vi "FGV_HoldingRegs.vi"(6 "FGV_enum":T3=enum."Read", 7 "unit ID":u8=1, 8 "error in (no error)":errorcluster, 9 "FGV_ data cluster":T1={"demux1_10(x6)_encode"=enum."demux1_10_channel0", "mux10_1(x6)_encode"=enum."mux10_1_channel0", "MB Relay01"=[FALSE, FALSE, FALSE, FALSE, FALSE, FALSE], "SpareRelays (DPDT)"=[], "mux6_1(3wires)_encode"=enum."mux6-1_channel0", "mux2-1(DMM I) encode"=enum."DMM I (0.5)", "5V enable"=FALSE, "SpareRelays (SPDT)"=[FALSE, FALSE, FALSE, FALSE, FALSE, FALSE, FALSE, FALSE, FALSE, FALSE, FALSE, FALSE, FALSE, FALSE, FALSE, FALSE, FALSE, FALSE, FALSE, FALSE, FALSE, FALSE, FALSE, FALSE, FALSE, FALSE, FALSE, FALSE, FALSE, FALSE, FALSE, FALSE], "JIG_RESET"=FALSE}, 10 "Instruments":T2=enum."mux10_1(x6)", 11 "Modbus master in":refnum<class "Modbus Master.lvclass">) -> (0 "error out":errorcluster, 2 "HoldingRegs":u16[](array[numeric]), 3 "Modbus master out":refnum<class "Modbus Master.lvclass">)   [LabVIEW 2018, in "MB Relay.lvlib"]
uses:
  MB Relay.lvlib
  type defs/FGV enum.ctl
  <vilib>/NI/Modbus Library/API/Master/Modbus Master.lvclass
  C:/Program Files (x86)/National Instruments/LabVIEW 2018/vi.lib/NI/Modbus Library/API/Modbus API.lvclass
  type defs/MB relays _InstrumentType.ctl
  type defs/FGV data cluster.ctl
  <vilib>/NI/Modbus Library/API/Modbus API.lvclass/Modbus API.ctl
  <vilib>/NI/Modbus Library/Transmission Data Unit/Transmission Data Unit.lvclass/Transmission Data Unit.ctl
  <vilib>/NI/Modbus Library/Transmission Data Unit/Write Unit ID.vi
  <vilib>/NI/Modbus Library/API/Read Transmission Data Unit.vi
  <vilib>/NI/Modbus Library/API/Write Transmission Data Unit.vi
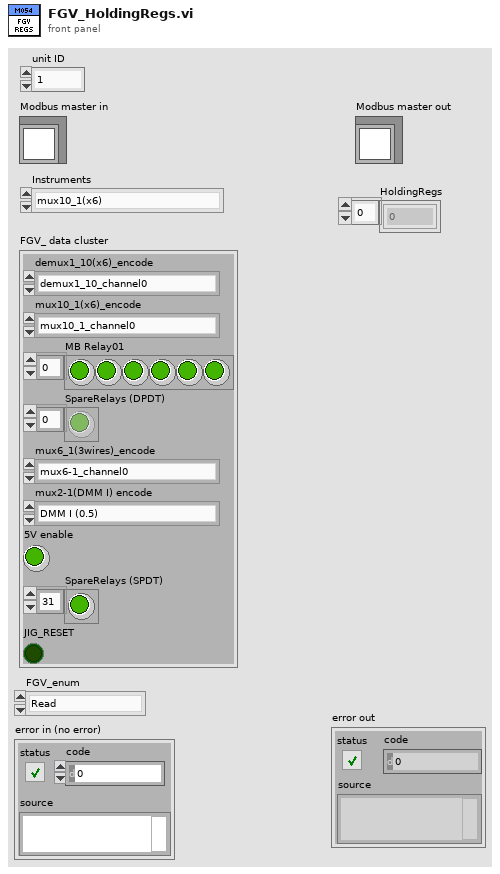
[diagram p1: front panel]
types:
  T1 = typedef "MB Relay.lvlib/FGV data cluster.ctl" = cluster{"demux1_10(x6)_encode":enum16{"demux1_10_channel0", "demux1_10_channel1", "demux1_10_channel2", "demux1_10_channel3", "demux1_10_channel4", "demux1_10_channel5", "demux1_10_channel6", "demux1_10_channel7", "demux1_10_channel8", "demux1_10_channel9", "demux1_10_channel10"}, "mux10_1(x6)_encode":enum16{"mux10_1_channel0", "mux10_1_channel1", "mux10_1_channel2", "mux10_1_channel3", "mux10_1_channel4", "mux10_1_channel5", "mux10_1_channel6", "mux10_1_channel7", "mux10_1_channel8", "mux10_1_channel9", "mux10_1_channel10"}, "MB Relay01":bool[], "SpareRelays (DPDT)":bool[], "mux6_1(3wires)_encode":enum16{"mux6-1_channel0", "mux6_1_channel1_0", "mux6_1_channel1_1", "mux6-1_channel1_2", "mux6_1_channel1_3", "mux6_1_channel2_0", "mux6_1_channel2_1", "mux6_1_channel2_2", "mux6_1_channel2_3", "mux6_1_channel3_0", "mux6_1_channel3_1", "mux6_1_channel3_2", "mux6_1_channel3_3", "mux6_1_channel4_0", "mux6_1_channel4_1", "mux6_1_channel4_2", "mux6_1_channel4_3", "mux6_1_channel5_0", "mux6_1_channel5_1", "mux6_1_channel5_2", "mux6_1_channel5_3", "mux6_1_channel6_0", "mux6_1_channel6_1", "mux6_1_channel6_2", "mux6_1_channel6_3"}, "mux2-1(DMM I) encode":enum16{"DMM I (0.5)", "DMM I (12)"}, "5V enable":bool, "SpareRelays (SPDT)":bool[], "JIG_RESET":bool}
  T2 = typedef "MB Relay.lvlib/MB relays _InstrumentType.ctl" = enum16{"JIG_TRIGGER", "JIG_RESET", "Relay SelfTest", "counter", "demux1_10(x6)", "mux10_1(x6)", "mux6_1(3wires)", "MB_Relay_01(eMICs)", "SpareRelays(DPDT)", "Optos", "Inputs", "DMM I 0.5", "SpareRelays (SPDT)", "SC enable"}
  T3 = typedef "MB Relay.lvlib/FGV enum.ctl" = enum16{"Write", "Init FGV", "Read", "All OFF", "All ON"}
  T4 = enum16{"demux1_10_channel0", "demux1_10_channel1", "demux1_10_channel2", "demux1_10_channel3", "demux1_10_channel4", "demux1_10_channel5", "demux1_10_channel6", "demux1_10_channel7", "demux1_10_channel8", "demux1_10_channel9", "demux1_10_channel10"}
  T5 = enum16{"mux10_1_channel0", "mux10_1_channel1", "mux10_1_channel2", "mux10_1_channel3", "mux10_1_channel4", "mux10_1_channel5", "mux10_1_channel6", "mux10_1_channel7", "mux10_1_channel8", "mux10_1_channel9", "mux10_1_channel10"}
  T6 = enum16{"mux6-1_channel0", "mux6_1_channel1_0", "mux6_1_channel1_1", "mux6-1_channel1_2", "mux6_1_channel1_3", "mux6_1_channel2_0", "mux6_1_channel2_1", "mux6_1_channel2_2", "mux6_1_channel2_3", "mux6_1_channel3_0", "mux6_1_channel3_1", "mux6_1_channel3_2", "mux6_1_channel3_3", "mux6_1_channel4_0", "mux6_1_channel4_1", "mux6_1_channel4_2", "mux6_1_channel4_3", "mux6_1_channel5_0", "mux6_1_channel5_1", "mux6_1_channel5_2", "mux6_1_channel5_3", "mux6_1_channel6_0", "mux6_1_channel6_1", "mux6_1_channel6_2", "mux6_1_channel6_3"}
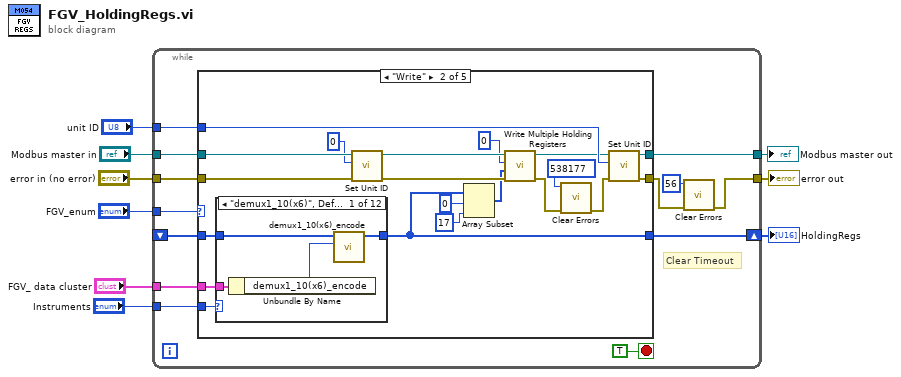
[diagram p0: block diagram]
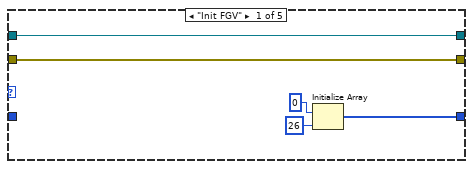
[diagram p2: hidden frame]
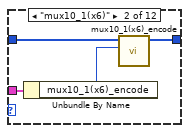
[diagram p3: hidden frame]
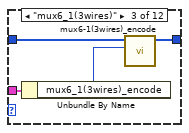
[diagram p4: hidden frame]
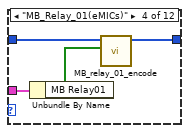
[diagram p5: hidden frame]
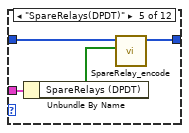
[diagram p6: hidden frame]
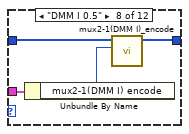
[diagram p9: hidden frame]
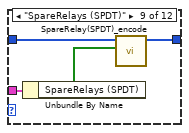
[diagram p10: hidden frame]
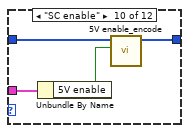
[diagram p11: hidden frame]
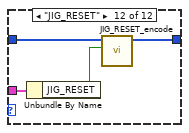
[diagram p13: hidden frame]
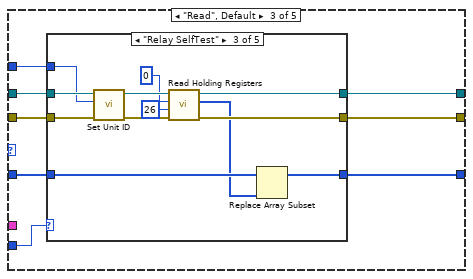
[diagram p14: hidden frame]
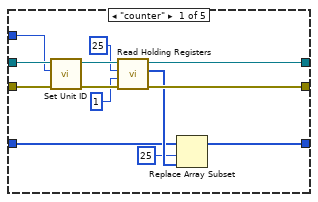
[diagram p15: hidden frame]
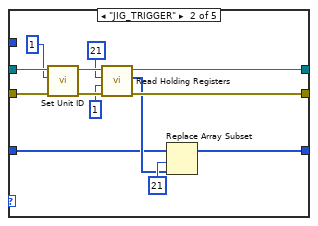
[diagram p16: hidden frame]
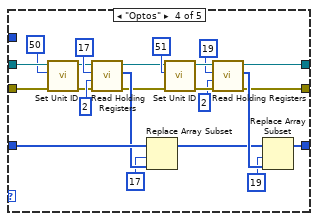
[diagram p17: hidden frame]
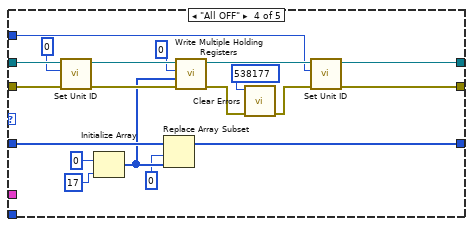
[diagram p19: hidden frame]
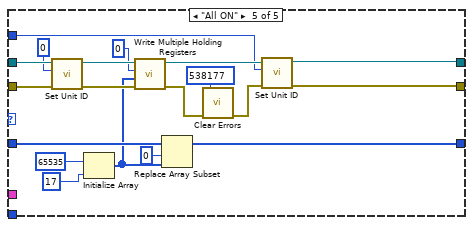
[diagram p20: hidden frame]
diagram:
  n1 = while {
    tunnel: "FGV_enum" -> [w21]
    shift-right: [w20] -> w4
    shift-left: _ -> [w11]
    tunnel: "error in (no error)" -> [w19]
    tunnel: [w14] -> w7
    tunnel: "Modbus master in" -> [w18]
    tunnel: [w17] -> w5
    tunnel: "unit ID" -> [w16]
    tunnel: "Instruments" -> [w12]
    tunnel: "FGV_ data cluster" -> [w10]
    stop <- TRUE stop-if-true
    # "Clear Timeout"
    n2 = case shown="\"Write\"" w21 {
      tunnel: [w24 w31 w91 w161 w184] -> w20
      tunnel: w19 -> [w27 w47 w94 w177 w194]
      tunnel: [w27 w37 w90 w166 w182] -> w15
      tunnel: w18 -> [w23 w44 w93 w175 w192]
      tunnel: [w23 w39 w89 w165 w180] -> w17
      tunnel: w16 -> [_ w36 w87 w164 w179]
      tunnel: w12 -> [_ w32 w88 _ _]
      tunnel: w11 -> [_ w29 w92 w163 w186]
      tunnel: w10 -> [_ w28 _ _ _]
      frame "Init FGV" {
        n3 = Initialize Array(u16 0, 26 ("dimension size")) -> (w24:u16[])
      }
      frame "Write" {
        n4 = case shown="\"demux1_10(x6)\", Default" w32 {
          tunnel: w29 -> [w51 w55 w57 w63 w67 w68 w69 w73 w77 w78 w82 w86]
          tunnel: [w50 w54 w58 w62 w66 w68 w69 w72 w76 w79 w82 w85] -> w31
          tunnel: w28 -> [w49 w53 w59 w61 w65 _ _ w71 w75 w81 _ w84]
          frame "demux1_10(x6)", Default {
            n5 = Unbundle By Name(w49) -> ("demux1_10(x6)_encode"=w48:T4)
            n6 = call "demux1_10(x6)_encode.vi"("demux1_10(x6)_encode"=w48, "Mem_mapping in"=w51) -> ("MemMapping Out"=w50:u16[])  [unwired: 8 in, 1 out]
          }
          frame "mux10_1(x6)" {
            n7 = Unbundle By Name(w53) -> ("mux10_1(x6)_encode"=w52:T5)
            n8 = call "mux10_1(x6)_encode.vi"("mux10_1(x6)_encode"=w52, "Mem_mapping in"=w55) -> ("MemMapping Out"=w54:u16[])  [unwired: 8 in, 1 out]
          }
          frame "mux6_1(3wires)" {
            n9 = Unbundle By Name(w59) -> ("mux6_1(3wires)_encode"=w56:T6)
            n10 = call "mux6-1(3wires)_encode.vi"("mux6_1(3wires)_encode"=w56, "Mem_mapping in"=w57) -> ("MemMapping Out"=w58:u16[])  [unwired: 8 in, 1 out]
          }
          frame "MB_Relay_01(eMICs)" {
            n11 = Unbundle By Name(w61) -> ("MB Relay01"=w60:bool[])
            n12 = call "MB_relay_01_encode.vi"("eMic1-6"=w60, "Mem_mapping in"=w63) -> ("MemMapping Out"=w62:u16[])  [unwired: 8 in, 1 out]
          }
          frame "SpareRelays(DPDT)" {
            n13 = Unbundle By Name(w65) -> ("SpareRelays (DPDT)"=w64:bool[])
            n14 = call "SpareRelay_encode.vi"("Array"=w64, "Mem_mapping in"=w67) -> ("MemMapping Out"=w66:u16[])  [unwired: 8 in, 1 out]
          }
          frame "Optos" {
          }
          frame "Inputs" {
          }
          frame "DMM I 0.5" {
            n15 = Unbundle By Name(w71) -> ("mux2-1(DMM I) encode"=w70:enum16{"DMM I (0.5)", "DMM I (12)"})
            n16 = call "mux2-1(DMM I)_encode.vi"("mux2-1(DMM I)"=w70, "Mem_mapping in"=w73) -> ("MemMapping Out"=w72:u16[])  [unwired: 8 in, 1 out]
          }
          frame "SpareRelays (SPDT)" {
            n17 = Unbundle By Name(w75) -> ("SpareRelays (SPDT)"=w74:bool[])
            n18 = call "SpareRelay(SPDT)_encode.vi"("data"=w74, "Mem_mapping in"=w77) -> ("MemMapping Out"=w76:u16[])  [unwired: 8 in, 1 out]
          }
          frame "SC enable" {
            n19 = Unbundle By Name(w81) -> ("5V enable"=w80:bool)
            n20 = call "5V enable_encode.vi"("5V enable"=w80, "Mem_mapping in"=w78) -> ("MemMapping Out"=w79:u16[])  [unwired: 8 in, 1 out]
          }
          frame "counter" {
          }
          frame "JIG_RESET" {
            n21 = Unbundle By Name(w84) -> ("JIG_RESET"=w83:bool)
            n22 = call "JIG_RESET_encode.vi"("JIG RESET"=w83, "Mem_mapping in"=w86) -> ("MemMapping Out"=w85:u16[])  [unwired: 8 in, 1 out]
          }
        }
        n23 = call <vilib>:"Set Unit ID.vi"("error in"=w47, "unit ID"=u8 0, "Modbus master in"=w44) -> ("error out"=w46:errorcluster, "Modbus master out"=w45:refnum<class "Modbus Master.lvclass">)  [unwired: 7 in]
        n24 = Array Subset(array=w31, index=0, length=17) -> (w33:u16[])
        n25 = call-dynamic "Write Multiple Holding Registers.vi"("error in"=w46, "registers to write"=w33, "starting address"=u16 0, "Modbus master in"=w45) -> ("error out"=w41:errorcluster, "Modbus master out"=w35:refnum<class "Modbus Master.lvclass">)  [unwired: 6 in]
        n26 = call <vilib>:"Clear Errors.vi"("error in (no error)"=w41, "specific error code to clear (0: all)"=538177) -> ("error out"=w38:errorcluster)  [unwired: 4 in, 1 out]
        n27 = call <vilib>:"Set Unit ID.vi"("error in"=w38, "unit ID"=w36, "Modbus master in"=w35) -> ("error out"=w37:errorcluster, "Modbus master out"=w39:refnum<class "Modbus Master.lvclass">)  [unwired: 7 in]
      }
      frame "Read", Default {
        n28 = case shown="\"Relay SelfTest\"" w88 {
          tunnel: w94 -> [w106 w115 w131 w153 w157]
          tunnel: w93 -> [w107 w116 w132 w150 w158]
          tunnel: w92 -> [w97 w110 w123 w149 w156]
          tunnel: [w96 w109 w122 w147 w156] -> w91
          tunnel: [w100 w113 w126 w137 w157] -> w90
          tunnel: [w99 w114 w127 w136 w158] -> w89
          tunnel: w87 -> [w105 _ w130 _ _]
          frame "counter" {
            n29 = call <vilib>:"Set Unit ID.vi"("error in"=w106, "unit ID"=w105, "Modbus master in"=w107) -> ("error out"=w103:errorcluster, "Modbus master out"=w104:refnum<class "Modbus Master.lvclass">)  [unwired: 7 in]
            n30 = call-dynamic "Read Holding Registers.vi"("error in"=w103, "number of inputs"=u16 1, "starting address"=u16 25, "Modbus master in"=w104) -> ("error out"=w100:errorcluster, "register values"=w98:u16[], "Modbus master out"=w99:refnum<class "Modbus Master.lvclass">)  [unwired: 5 in]
            n31 = Replace Array Subset(array=w97, new element=w98, index=25) -> (w96:u16[])
          }
          frame "JIG_TRIGGER" {
            n32 = call <vilib>:"Set Unit ID.vi"("error in"=w115, "unit ID"=u8 1 ("number of inputs"), "Modbus master in"=w116) -> ("error out"=w119:errorcluster, "Modbus master out"=w120:refnum<class "Modbus Master.lvclass">)  [unwired: 7 in]
            n33 = call-dynamic "Read Holding Registers.vi"("error in"=w119, "number of inputs"=u16 1, "starting address"=u16 21, "Modbus master in"=w120) -> ("error out"=w113:errorcluster, "register values"=w111:u16[], "Modbus master out"=w114:refnum<class "Modbus Master.lvclass">)  [unwired: 5 in]
            n34 = Replace Array Subset(array=w110, new element=w111, index=21) -> (w109:u16[])
          }
          frame "Relay SelfTest" {
            n35 = call <vilib>:"Set Unit ID.vi"("error in"=w131, "unit ID"=w130, "Modbus master in"=w132) -> ("error out"=w129:errorcluster, "Modbus master out"=w128:refnum<class "Modbus Master.lvclass">)  [unwired: 7 in]
            n36 = call-dynamic "Read Holding Registers.vi"("error in"=w129, "number of inputs"=u16 26, "starting address"=u16 0, "Modbus master in"=w128) -> ("error out"=w126:errorcluster, "register values"=w121:u16[], "Modbus master out"=w127:refnum<class "Modbus Master.lvclass">)  [unwired: 5 in]
            n37 = Replace Array Subset(array=w123, new element=w121) -> (w122:u16[])  [unwired: 1 in]
          }
          frame "Optos" {
            n38 = call <vilib>:"Set Unit ID.vi"("error in"=w153, "unit ID"=u8 50, "Modbus master in"=w150) -> ("error out"=w152:errorcluster, "Modbus master out"=w151:refnum<class "Modbus Master.lvclass">)  [unwired: 7 in]
            n39 = call-dynamic "Read Holding Registers.vi"("error in"=w152, "number of inputs"=u16 2, "starting address"=u16 17, "Modbus master in"=w151) -> ("error out"=w140:errorcluster, "register values"=w148:u16[], "Modbus master out"=w139:refnum<class "Modbus Master.lvclass">)  [unwired: 5 in]
            n40 = Replace Array Subset(array=w149, new element=w148, index=17) -> (w135:u16[])
            n41 = call <vilib>:"Set Unit ID.vi"("error in"=w140, "unit ID"=u8 51, "Modbus master in"=w139) -> ("error out"=w143:errorcluster, "Modbus master out"=w144:refnum<class "Modbus Master.lvclass">)  [unwired: 7 in]
            n42 = call-dynamic "Read Holding Registers.vi"("error in"=w143, "number of inputs"=u16 2, "starting address"=u16 19, "Modbus master in"=w144) -> ("error out"=w137:errorcluster, "register values"=w138:u16[], "Modbus master out"=w136:refnum<class "Modbus Master.lvclass">)  [unwired: 5 in]
            n43 = Replace Array Subset(array=w135, new element=w138, index=19) -> (w147:u16[])
          }
          frame "Inputs", Default {
          }
        }
      }
      frame "All OFF" {
        n44 = call <vilib>:"Set Unit ID.vi"("error in"=w177, "unit ID"=u8 0, "Modbus master in"=w175) -> ("error out"=w176:errorcluster, "Modbus master out"=w174:refnum<class "Modbus Master.lvclass">)  [unwired: 7 in]
        n45 = Initialize Array(u16 0, 17 ("dimension size")) -> (w162:u16[])
        n46 = Replace Array Subset(array=w163, new element=w162, index=0) -> (w161:u16[])
        n47 = call-dynamic "Write Multiple Holding Registers.vi"("error in"=w176, "registers to write"=w162, "starting address"=u16 0, "Modbus master in"=w174) -> ("error out"=w172:errorcluster, "Modbus master out"=w167:refnum<class "Modbus Master.lvclass">)  [unwired: 6 in]
        n48 = call <vilib>:"Clear Errors.vi"("error in (no error)"=w172, "specific error code to clear (0: all)"=538177) -> ("error out"=w168:errorcluster)  [unwired: 4 in, 1 out]
        n49 = call <vilib>:"Set Unit ID.vi"("error in"=w168, "unit ID"=w164, "Modbus master in"=w167) -> ("error out"=w166:errorcluster, "Modbus master out"=w165:refnum<class "Modbus Master.lvclass">)  [unwired: 7 in]
      }
      frame "All ON" {
        n50 = call <vilib>:"Set Unit ID.vi"("error in"=w194, "unit ID"=u8 0, "Modbus master in"=w192) -> ("error out"=w193:errorcluster, "Modbus master out"=w191:refnum<class "Modbus Master.lvclass">)  [unwired: 7 in]
        n51 = Initialize Array(u16 65535, 17 ("dimension size")) -> (w185:u16[])
        n52 = call-dynamic "Write Multiple Holding Registers.vi"("error in"=w193, "registers to write"=w185, "starting address"=u16 0, "Modbus master in"=w191) -> ("error out"=w189:errorcluster, "Modbus master out"=w181:refnum<class "Modbus Master.lvclass">)  [unwired: 6 in]
        n53 = Replace Array Subset(array=w186, new element=w185, index=0) -> (w184:u16[])
        n54 = call <vilib>:"Clear Errors.vi"("error in (no error)"=w189, "specific error code to clear (0: all)"=538177) -> ("error out"=w183:errorcluster)  [unwired: 4 in, 1 out]
        n55 = call <vilib>:"Set Unit ID.vi"("error in"=w183, "unit ID"=w179, "Modbus master in"=w181) -> ("error out"=w182:errorcluster, "Modbus master out"=w180:refnum<class "Modbus Master.lvclass">)  [unwired: 7 in]
      }
    }
    n56 = call <vilib>:"Clear Errors.vi"("error in (no error)"=w15, "specific error code to clear (0: all)"=56) -> ("error out"=w14:errorcluster)  [unwired: 4 in, 1 out]
  }
  "error out" <- w7
  "Modbus master out" <- w5
  "HoldingRegs" <- w4
